vi "proj_dtrnd (SubVI).vi"(9 "Trend":dbl, 10 "N_packets":dbl=7.0, 11 "String":string="E:\\Ankur\\MATLAB\\Auto_Scan_reconst\\Perf_test_Video\\1_1.txt") -> (0 "error out":errorcluster, 3 "Real":dbl)   [LabVIEW 2018]
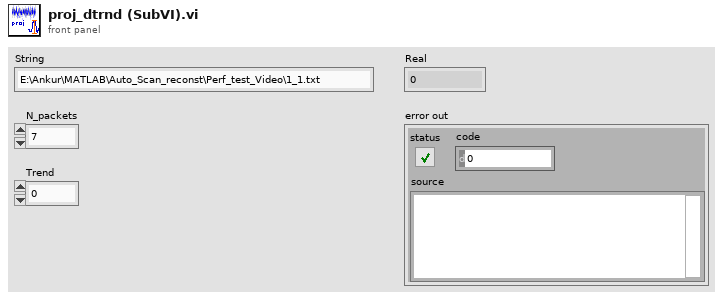
[diagram p1: front panel]
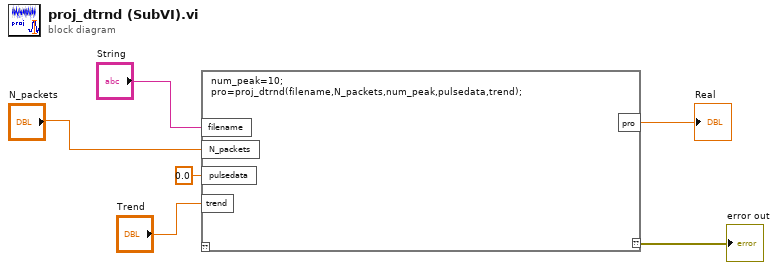
[diagram p0: block diagram]
diagram:
  n1 = script code="num_peak=10;\npro=proj_dtrnd(filename,N_packets,num_peak,pulsedata,trend);"("filename"="String", "N_packets"="N_packets", "trend"="Trend", "pulsedata"=0.0 ("Real")) -> ("??"=→"error out":errorcluster, "pro"=→"Real":dbl)  [unwired: 1 in]
